vi "Firmware Version.vi"(8 "error in (no error)":errorcluster, 11 "EPU452 in":refnum<class "EPU452.lvclass">) -> (0 "error out":errorcluster, 1 "Version":string, 2 "Response":string, 3 "EPU452 out":refnum<class "EPU452.lvclass">)   [LabVIEW 2018, in "EPU452.lvclass"]
uses:
  EPU452.lvclass
  <vilib>/regexp/Match Regular Expression.xnode
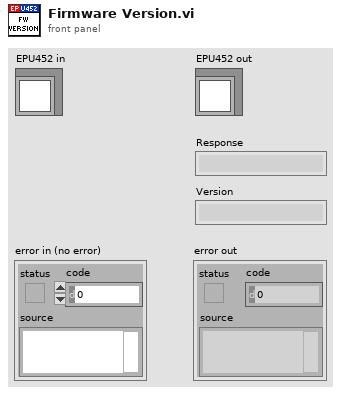
[diagram p1: front panel]
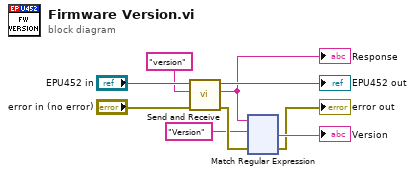
[diagram p0: block diagram]
diagram:
  n1 = call "Send and Receive.vi"("error in (no error)"="error in (no error)", "Command"="version", "EPU452 in"="EPU452 in") -> ("error out"=w8:errorcluster, "Response"=w5:string, "EPU452 out"=→"EPU452 out":refnum<class "EPU452.lvclass">)  [unwired: 6 in]
  "Response" <- w5
  n2 = xnode "Match Regular Expression"("input string"=w5, "regular expression"="Version" ("format string"), "error in"=w8) -> ("after match"=→"Version":string, "error out"=→"error out":errorcluster)  [unwired: 3 in, 3 out]
